vi "analyseImage.vi"(8 "error in (no error)":errorcluster, 10 "Array":T1(array[cluster]), 11 "AbsorptionAnalyser in":refnum<class "AbsorptionAnalyser.lvclass">) -> (0 "error out":errorcluster, 3 "AbsorptionAnalyser out":refnum<class "AbsorptionAnalyser.lvclass">)   [LabVIEW 2011, in "Tools.lvlib" / "Imaging.lvlib" / "AbsorptionAnalyser.lvclass"]
uses:
  AbsorptionAnalyser.lvclass
  Filing/FileNeologist/FileNeologist.lvclass
  ImageAnalyser.lvclass
  Filing/FileSystem/FileSystem.lvclass
  Imaging.lvlib
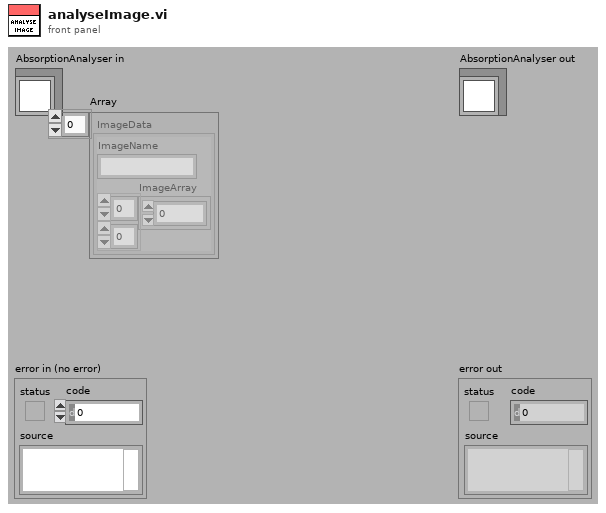
[diagram p1: front panel]
types:
  T1 = cluster{"ImageName":string, "ImageArray":sgl[][]}[]
  T2 = cluster{"Name":string, "Results":dbl[], "AnalysisType":string}
  T3 = cluster{"Left":i32, "Top":i32, "Right":i32, "Bottom":i32}
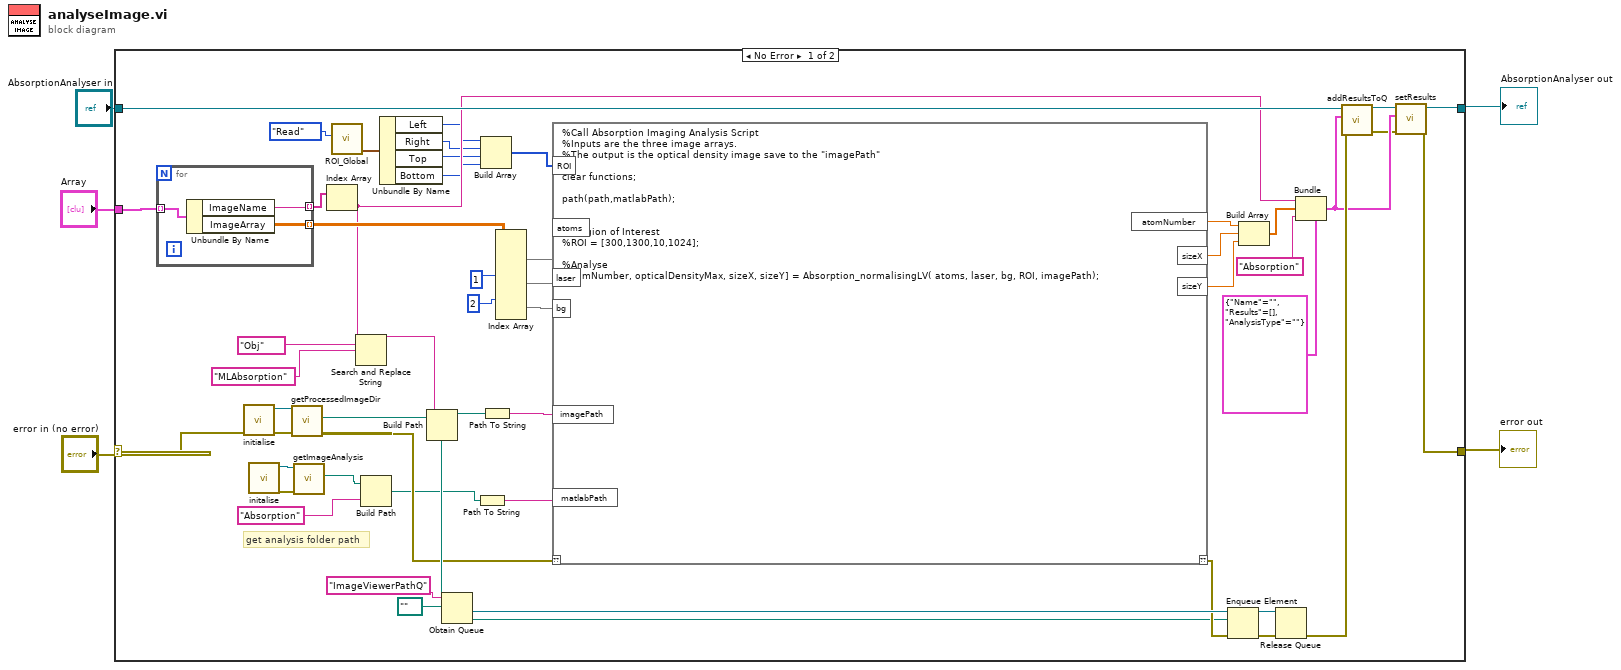
[diagram p0: block diagram]
diagram:
  n1 = case shown="No Error" "error in (no error)" {
    selector: "error in (no error)" -> [w29 w61]
    tunnel: [w17 w61] -> w4
    tunnel: [w20 w60] -> w2
    tunnel: "AbsorptionAnalyser in" -> [w55 w60]
    tunnel: "Array" -> [w54 _]
    frame No Error {
      # "get analysis folder path"
      n2 = for {
        tunnel: w54 -> [w59] mode=indexing
        tunnel: [w58] -> w53 mode=indexing
        tunnel: [w57] -> w49 mode=indexing
        n3 = Unbundle By Name(w59) -> ("ImageName"=w57:string, "ImageArray"=w58:sgl[][])
      }
      n4 = call "initialise.vi"("error in (no error)"=w29) -> ("error out"=w45:errorcluster, "FileNeologist out"=w46:refnum<class "FileNeologist.lvclass">)  [unwired: 9 in]
      n5 = call "initalise.vi"() -> ("error out"=w25:errorcluster, "FileSystem out"=w26:refnum<class "FileSystem.lvclass">)  [unwired: 10 in]
      n6 = call-dynamic "getProcessedImageDir.vi"("error in (no error)"=w45, "FileNeologist in"=w46) -> ("error out"=w28:errorcluster, "Path"=w44:path)  [unwired: 7 in, 1 out]
      n7 = call "getImageAnalysis.vi"("error in (no error)"=w25, "FileSystem in"=w26) -> ("ImageAnalysis"=w24:path)  [unwired: 7 in, 2 out]
      n8 = Index Array(array=w49) -> (element=w32:string)  [unwired: 1 in]
      n9 = call "ROI_Global.vi"("Action"=enum16{"Write", "Read"}."Read") -> ("ROI"=w12:T3)  [unwired: 10 in]
      n10 = Search and Replace String(input string=w32, search string="Obj", replace string="MLAbsorption") -> (result string=w43:string)  [unwired: 5 in, 3 out]
      n11 = Build Path(base path=w24, name or relative path="Absorption") -> (appended path=w22:path)
      n12 = Unbundle By Name(w12) -> ("Left"=w10:i32, "Right"=w9:i32, "Top"=w8:i32, "Bottom"=w7:i32)
      n13 = Build Path(base path=w44, name or relative path=w43) -> (appended path=w35:path)
      n14 = Obtain Queue(name (unnamed)="ImageViewerPathQ", element data type=path "") -> (queue out=w40:refnum<queue>)  [unwired: 3 in, 2 out]
      n15 = Path To String(path=w22) -> (string=w27:string)
      n16 = Build Array(w10, w9, w8, w7) -> (w11:i32[])
      n17 = Path To String(path=w35) -> (string=w37:string)
      n18 = Index Array(array=w53, index (dim 0) #2=1, index (dim 0) #3=2) -> (element #1=w13:sgl[][], element #2=w51:sgl[][], element #3=w50:sgl[][])  [unwired: 7 in]
      n19 = script code="%Call Absorption Imaging Analysis Script \n%Inputs are the three image arrays.\n%The output is the optical density image save to the \"imagePath\"\n\nclear functions;\n\npath(path,matlabPath);\n\n\n% Region of Interest\n%ROI = [300,1300,10,1024];\n\n%Analyse\n[atomNumber, opticalDensityMax, sizeX, sizeY] = Absorption_normalisingLV( atoms, laser, bg, ROI, imagePath);"("??"=w28, "bg"=w50, "laser"=w51, "atoms"=w13, "imagePath"=w37, "matlabPath"=w27, "ROI"=w11) -> ("??"=w36:errorcluster, "atomNumber"=w16:dbl, "sizeX"=w15:dbl, "sizeY"=w14:dbl)
      n20 = Enqueue Element(queue=w40, element=w35, error in (no error)=w36) -> (queue out=w39:refnum<queue>, error out=w38:errorcluster)  [unwired: 1 in, 1 out]
      n21 = Build Array(w16, w15, w14) -> (w33:dbl[])
      n22 = Release Queue(queue=w39, error in (no error)=w38) -> (error out=w34:errorcluster)  [unwired: 1 in, 2 out]
      n23 = Bundle(cluster=T2 {"Name"="", "Results"=[], "AnalysisType"=""} ("output cluster"), "Name"=w32, "Results"=w33, "AnalysisType"="Absorption") -> (w19:T2)
      n24 = call "addResultsToQ.vi"("error in (no error)"=w34, "Results"=w19, "ImageAnalyser in"=w55) -> ("error out"=w18:errorcluster, "ImageAnalyser out"=w21:refnum<class "AbsorptionAnalyser.lvclass">)  [unwired: 7 in]
      n25 = call "setResults.vi"("error in (no error)"=w18, "results"=w19, "ImageAnalyser in"=w21) -> ("error out"=w17:errorcluster, "ImageAnalyser out"=w20:refnum<class "AbsorptionAnalyser.lvclass">)  [unwired: 7 in]
    }
    frame Error {
    }
  }
  "error out" <- w4
  "AbsorptionAnalyser out" <- w2
